vi "Thermo_sendsignal.vi"(8 "error in (no error)":errorcluster, 10 "write buffer":string, 11 "VISA resource name":refnum<visa-resource-name>) -> (0 "error out":errorcluster, 3 "VISA resource name out":refnum<visa-resource-name>)   [LabVIEW 2015]
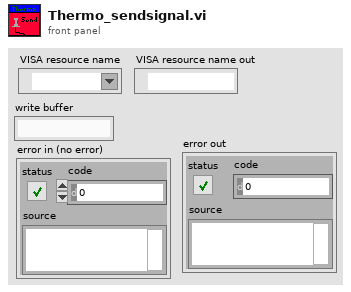
[diagram p1: front panel]
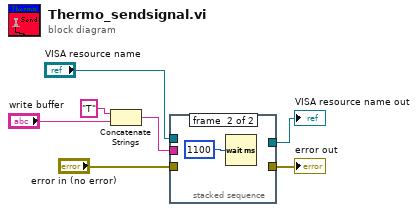
[diagram p0: block diagram]
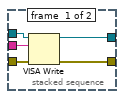
[diagram p2: hidden frame]
diagram:
  n1 = Concatenate Strings("T", "write buffer") -> (w3:string)
  n2 = stacked-sequence {
    tunnel: [w12 _] -> w5
    tunnel: [w11 _] -> w4
    tunnel: w3 -> [w10 _]
    tunnel: "VISA resource name" -> [w9 _]
    tunnel: "error in (no error)" -> [w8 _]
    frame #0 {
      n3 = VISA Write(VISA resource name=w9, write buffer=w10, error in (no error)=w8) -> (VISA resource name out=w12:refnum<visa-resource-name>, error out=w11:errorcluster)  [unwired: 1 out]
    }
    frame #1 {
      n4 = Wait (ms)(milliseconds to wait=u32 1100) -> ()  [unwired: 1 out]
    }
  }
  "VISA resource name out" <- w5
  "error out" <- w4
